vi "SystemController.GetDependencies.vi"(8 "error in (no error)":errorcluster, 11 "SystemController":refnum<class "SystemController.lvclass">) -> (0 "error out":errorcluster, 2 "Dependencies":T1, 3 "SystemController out":refnum<class "SystemController.lvclass">)   [LabVIEW 2017, in "SystemController.lvclass"]
doc: "---------------------------------------------------------------\nJKI State Machine Objects™\nhttp://jki.net/state-machine-objects/\nCopyright (C) 2005-2015, JKI <info@jki.net>\nALL RIGHTS RESERVEDJKI State Machine Objects (SMO) 1.0.0.5\nJKI - JKI\nCopyright (c) 2016, JKI"
uses:
  SystemController.lvclass
  Typedefs/Dependencies--Cluster.ctl
  Camera/Camera_class/Camera.lvclass
  ImageFacialDetection_class/ImageFacialDetection.lvclass
  SystemController.lvclass/SystemController.ctl
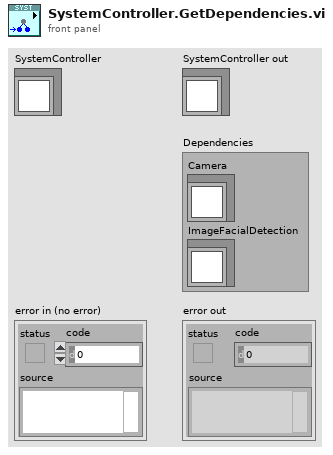
[diagram p1: front panel]
types:
  T1 = typedef "SystemController.lvclass/Dependencies--Cluster.ctl" = cluster{"Camera":refnum<class "Camera.lvclass">, "ImageFacialDetection":refnum<class "ImageFacialDetection.lvclass">}
  T2 = typedef "SystemController.lvclass/PrivateData--Ref.ctl" = refnum<data-value>
  T3 = typedef "SystemController.lvclass/PrivateData--Cluster.ctl" = cluster{"Configuration":T4, "Dependencies":T1, "ProcessedImage":T8, "Public Events":T9}
  T4 = typedef "SystemController.lvclass/Configuration--Cluster.ctl" = cluster{"Camera":T5, "Find Eyes":bool, "Acquisition Rate (ms)":i32}
  T5 = typedef "SystemController.lvclass/CameraConfig--Cluster.ctl" = cluster{"Simulate Camera":bool, "IMAQ Camera":T6, "Simulated Camera Image":path}
  T6 = typedef "Camera_IMAQdx.lvclass/Configuration--Cluster.ctl" = cluster{"Camera Interface Name":string, "Number of Buffers":u32, "Image Name":string, "Image Type":T7}
  T7 = typedef "Image Type" = u32
  T8 = typedef "IMAQ Image.ctl" = refnum<image>
  T9 = typedef "SystemController.lvclass/PublicEvents--Cluster.ctl" = cluster{"UIClosed":refnum<user-event>}
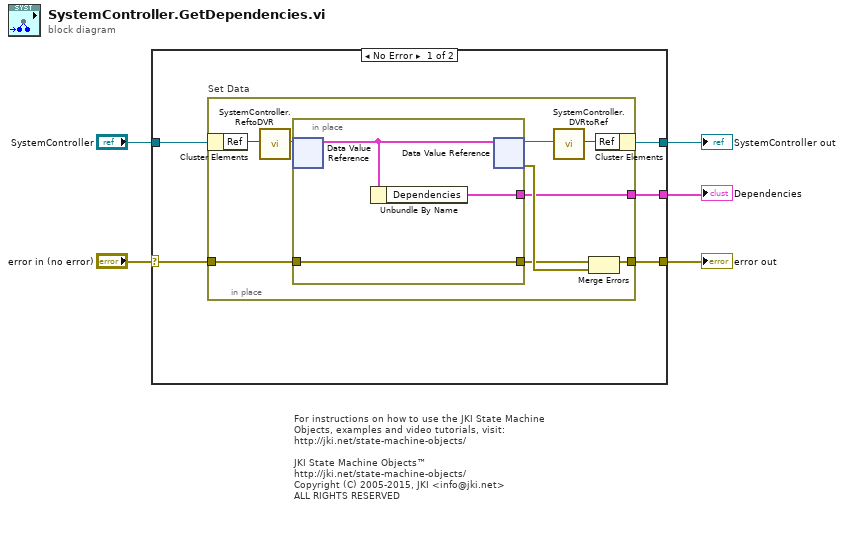
[diagram p0: block diagram]
diagram:
  # "For instructions on how to use the JKI State Machine Objects, examples and video tutorials, visit:\nhttp://jki.net/state-machine-objects/\n\nJKI State Machine Objects™\nhttp://jki.net/state-machine-objects/\nCopyright (C) 2005-2015, JKI <info@jki.net>\nALL RIGHTS RESERVED"
  n1 = case shown="No Error" "error in (no error)" {
    selector: "error in (no error)" -> [w9 w23]
    tunnel: "SystemController" -> [w10 w24]
    tunnel: [w8 w23] -> w4
    tunnel: [w7 w24] -> w3
    tunnel: [w6 _] -> w1
    frame No Error {
      n2 = in-place "Set Data" {
        in-place-border: w9 -> [w19]
        in-place-border: [w16] -> w8
        in-place-border: [w11] -> w6
        n3 = in-place-cluster #1(w10) -> ("Ref"=w15:u32)
        n4 = call "SystemController.ReftoDVR.vi"("Ref"=w15) -> ("Ref"=w14:T2)  [unwired: 10 in]
        n5 = in-place {
          in-place-border: w19 -> [w22]
          in-place-border: [w22] -> w17
          in-place-border: [w20] -> w11
          n6 = in-place-dvr #2(w14) -> (w21:T3)  [unwired: 1 out]
          n7 = Unbundle By Name(w21) -> ("Dependencies"=w20:T1)
          n8 = in-place-dvr #2(w21) -> (w13:T2, w18:errorcluster)
        }
        n9 = call "SystemController.DVRtoRef.vi"("Ref"=w13) -> ("Ref"=w12:u32)  [unwired: 10 in]
        n10 = Merge Errors(w17, w18) -> (w16:errorcluster)
        n11 = in-place-cluster #1("Ref"=w12) -> (w7:refnum<class "SystemController.lvclass">)
      }
    }
    frame Error {
    }
  }
  "error out" <- w4
  "SystemController out" <- w3
  "Dependencies" <- w1
